vi "SE_HV200.ProcDestructor.vi"(0 "i ref in":refnum<vi>, 3 "ms timeout (100)":i32=100, 5 "error in (no error)":errorcluster) -> (14 "i ref out":refnum<vi>, 17 "timed out":bool, 19 "error out":errorcluster)   [LabVIEW 2014, in "SE_HV200.lvlib"]
doc: "This is the counterpart to ProcConstructor and is called befor the \"deactivate\" is called. This can be used to shutdown/deinitialize things."
uses:
  SE_HV200.lvlib
  CS_Core/BaseProcess/BaseProcess.lvlib
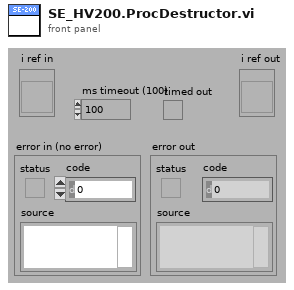
[diagram p1: front panel]
types:
  T1 = typedef "BaseProcess.lvlib/BaseProcess.i attribute.ctl" = cluster{"EventStatus":string, "EventError":i32, "PresetEvtWatchD":i32, "PresetPdcWatchD":i32, "EventTimeout":i32, "PeriodicInterval":i32, "Interface":string[], "Address":string[], "Special":string[], "PeriodicError":i32, "PeriodicStatus":string, "SuperProc":string, "Descriptors":T2[], "CaseRef":refnum<vi>, "PdcRef":refnum<vi>, "Thread Ref":refnum<vi>, "eventErrorID":i32, "eventStatusID":i32, "periodicErrorID":i32, "periodicStatusID":i32, "pdcCtrID":i32}
  T2 = typedef "BaseProcess.lvlib/BaseProcess.descriptor definition.ctl" = cluster{"selector":string, "descriptor":T3}
  T3 = typedef "BaseProcess.lvlib/BaseProcess.descriptor string definition.ctl" = string
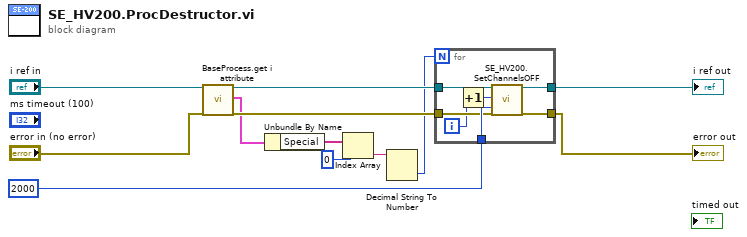
[diagram p0: block diagram]
diagram:
  n1 = call "BaseProcess.get i attribute.vi"("i ref in"="i ref in", "error in (no error)"="error in (no error)") -> ("i ref out"=w7:refnum<vi>, "i attribute"=w5:T1, "error out"=w6:errorcluster)  [unwired: 15 in]
  n2 = Unbundle By Name(w5) -> ("Special"=w4:string[])
  n3 = Index Array(array=w4, index=0) -> (element=w2:string)
  n4 = Decimal String To Number(string=w2) -> (number=w1:i32)  [unwired: 2 in, 1 out]
  n5 = for {
    N: w1 -> [_]
    tunnel: [w19] -> w12
    tunnel: [w18] -> w11
    tunnel: 2000 -> [w17]
    tunnel: w7 -> [w16]
    tunnel: w6 -> [w15]
    i -> [w14]
    n6 = Increment(x=w14) -> (x+1=w13:i32)
    n7 = call "SE_HV200.SetChannelsOFF.vi"("i ref in"=w16, "Channel"=w13, "Time out"=w17, "error in (no error)"=w15) -> ("i ref out"=w19:refnum<vi>, "error out"=w18:errorcluster)  [unwired: 13 in, 1 out]
  }
  "error out" <- w11
  "i ref out" <- w12
